vi "Get ATM Message.vi"(8 "error in (no error)":errorcluster, 11 "ATM View Model in":refnum<class "ATM View Model.lvclass">) -> (0 "error out":errorcluster, 2 "Message":string, 3 "ATM View Model out":refnum<class "ATM View Model.lvclass">)   [LabVIEW 2020, in "ATM View Model.lvclass"]
uses:
  ATM View Model.lvclass
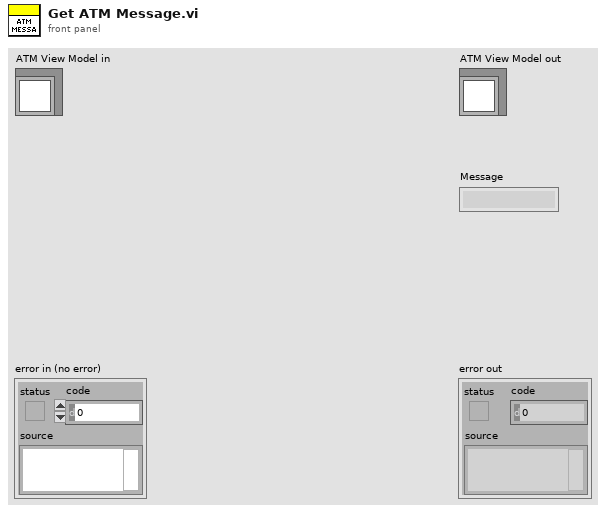
[diagram p1: front panel]
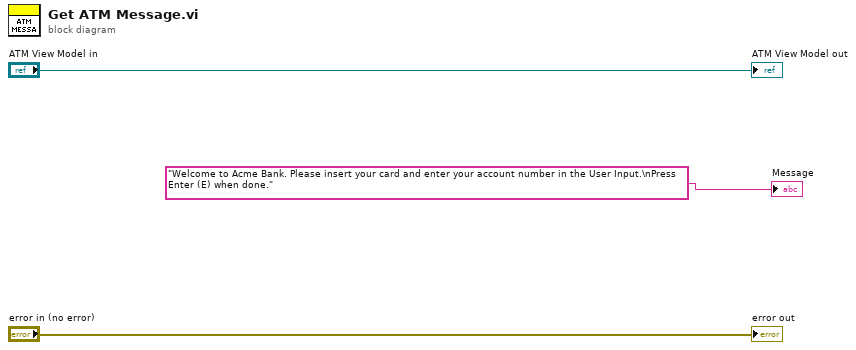
[diagram p0: block diagram]
diagram:
  "error out" <- "error in (no error)"
  "ATM View Model out" <- "ATM View Model in"
  "Message" <- "Welcome to Acme Bank. Please insert your card and enter your account number in the User Input.\nPress Enter (E) when done." ("Message")
